vi "RTSystemsCheck (1).vi"(8 "error in":errorcluster) -> (0 "error out":errorcluster)   [LabVIEW 2017]
uses:
  <vilib>/Platform/TimedLoop/XDataNode/timing_clust.ctl
  <vilib>/Platform/TimedLoop/XDataNode/nitl_modes.ctl
  <vilib>/Platform/TimedLoop/XDataNode/wakeup.ctl
  LoopPeriodGLOBAL.vi
  <vilib>/Platform/TimedLoop/XDataNode/loadnilvce.vi
  RTControl/StopGLOBAL.vi
  <vilib>/platform/TimedLoop/XDataNode/XDataNode.xnode
  <vilib>/Platform/TimedLoop/XDataNode/XDNodeRunTimeDep.lvlib
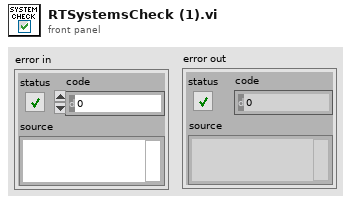
[diagram p1: front panel]
types:
  T1 = typedef "XDNodeRunTimeDep.lvlib/timing_clust.ctl" = cluster{"Expected End [f-1]":u64, "Actual End [f-1]":u64, "Finished Late? [f-1]":bool, "Expected End [i-1]":u64, "Actual End [i-1]":u64, "Finished Late? [i-1]":bool, "Expected Start [i]":u64, "Actual Start [i]":u64, "Expected Start [f]":u64, "Actual Start [f]":u64, "Source Name":string, "Structure Name":string, "Period":i64, "Deadline":i64, "Offset":i64, "Start":i64, "Priority":i32, "Timeout":i32, "Mode":T2, "Wakeup Reason":T3, "Error":errorcluster, "Source Type":string, "Secondary Source Type":string, "Global End Time":u64, "Global Start Time":u64, "Frame Duration":u64, "Iteration Duration":u64, "Assigned CPU":i32, "I/O Scan Engine Mode":u32}
  T2 = typedef "XDNodeRunTimeDep.lvlib/nitl_modes.ctl" = enum32{"No Change", "Process missed periods, maintain original phase", "Discard missed periods, maintain original phase", "Process missed periods, ignore original phase", "Discard missed periods, ignore original phase"}
  T3 = typedef "XDNodeRunTimeDep.lvlib/wakeup.ctl" = enum32{"Normal", "Aborted", "Asynchronous wakeup", "Timing source error", "Timed loop error", "Timeout"}
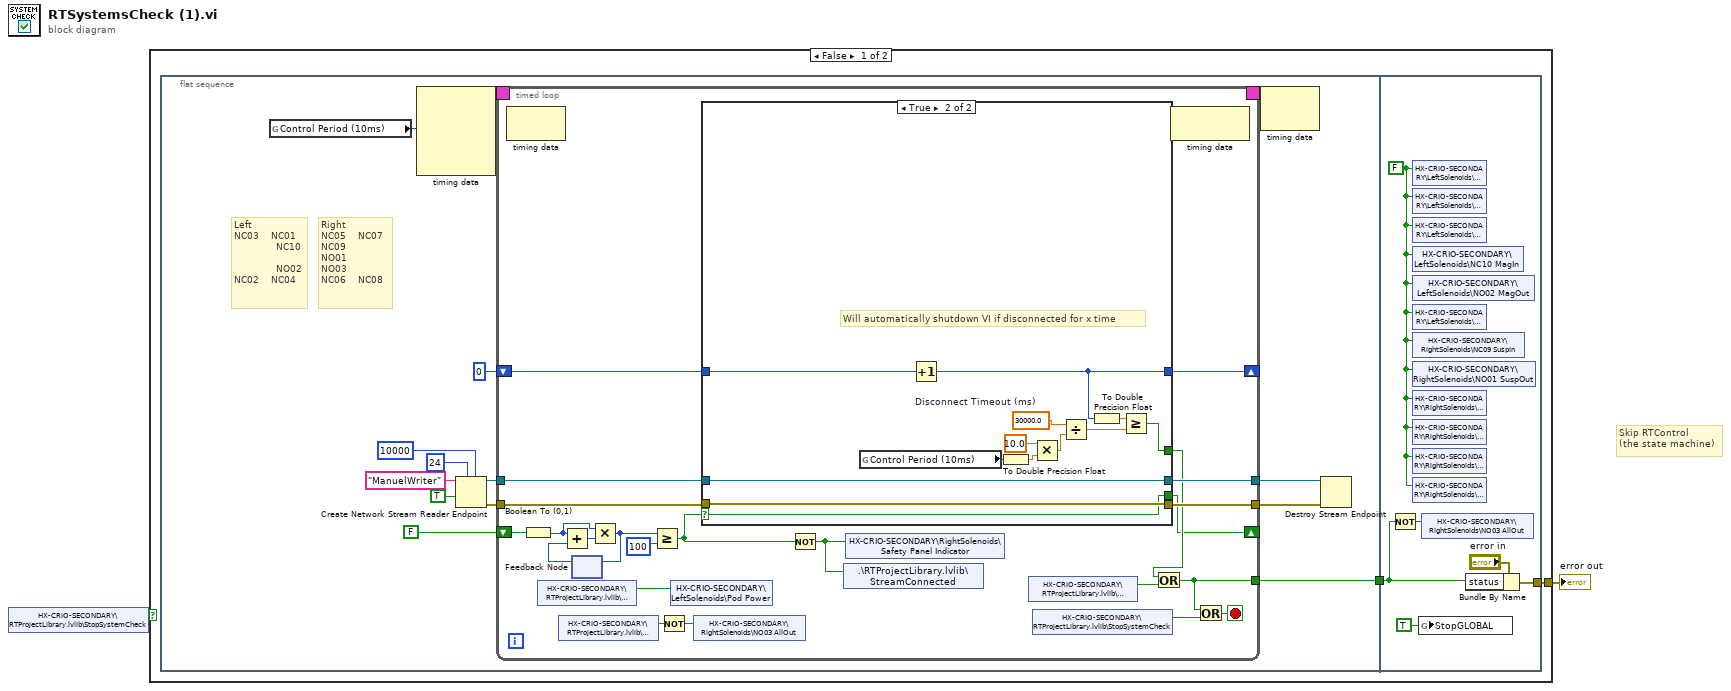
[diagram p0: block diagram]
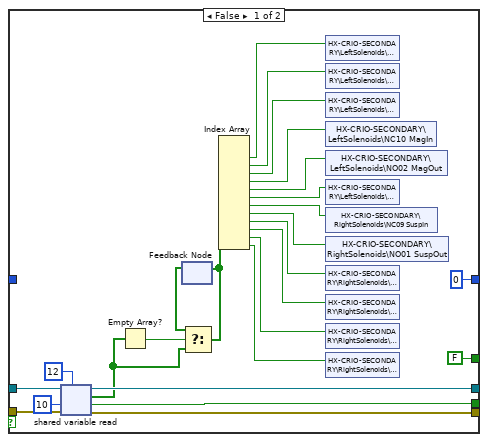
[diagram p2: hidden frame]
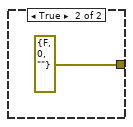
[diagram p3: hidden frame]
diagram:
  # "Skip RTControl\n(the state machine)"
  n1 = shared-variable "HX-CRIO-SECONDARY\\RTProjectLibrary.lvlib\\StopSystemCheck"() -> (w2:bool)  [unwired: 1 in, 1 out]
  n2 = case shown="False" w2 {
    tunnel: [w3 errorcluster {"status"=FALSE, "code"=0, "source"=""} ("error in")] -> w1
    frame False {
      n3 = flat-sequence {
        tunnel: [w7] -> w4
        tunnel: [w89] -> w3
        tunnel: w4 -> [w86]
        frame #0 {
          # "Right\nNC05    NC07\nNC09\nNO01\nNO03\nNC06    NC08"
          # "Left\nNC03    NC01\n              NC10\n\n              NO02\nNC02    NC04"
          n4 = global read "LoopPeriodGLOBAL.vi" "Control Period (10ms)"() -> (w16:i64)
          n5 = node-c288(w16) -> (w18:T1)  [unwired: 3 in]
          n6 = Create Network Stream Reader Endpoint(5:10000 ("timeout in ms (-1)"), 7:24 ("reader buffer size"), 9:TRUE, 11:"ManuelWriter" ("reader name")) -> (0:w14:errorcluster, 3:w15:refnum<k21>)  [unwired: 3 in]
          n7 = timed-loop {
            timing: w18 -> [_]
            timing-out: [_] -> w17
            tunnel: w15 -> [w30]
            tunnel: w14 -> [w29]
            tunnel: [w39] -> w10
            tunnel: [w38] -> w11
            shift-right: [w34] -> _
            shift-left: u16 0 -> [w35]
            tunnel: [w33] -> w7
            shift-right: [w27] -> _
            shift-left: FALSE -> [w25]
            stop <- w40 stop-if-true
            n8 = node-c288() -> ()  [unwired: 1 in, 1 out]
            n9 = Boolean To (0,1)(Boolean=w25) -> (0, 1=w23:i16)
            n10 = shared-variable "HX-CRIO-SECONDARY\\RTProjectLibrary.lvlib\\PodPower"() -> (w28:bool)  [unwired: 1 in, 1 out]
            n11 = shared-variable "HX-CRIO-SECONDARY\\RTProjectLibrary.lvlib\\VentTanks"() -> (w32:bool)  [unwired: 1 in, 1 out]
            n12 = feedback #1() -> (w22:i16)  [unwired: 1 in]
            n13 = Add(x=w23, y=w22) -> (x+y=w24:i16)
            n14 = Multiply(x=w23, y=w24) -> (x*y=w21:i16)
            n15 = feedback-in #1(w21) -> ()
            n16 = Greater Or Equal?(x=w21, y=i16 100) -> (x >= y?=w19:bool)
            n17 = Not(x=w32) -> (.not. x?=w31:bool)
            n18 = shared-variable "HX-CRIO-SECONDARY\\LeftSolenoids\\Pod Power"(w28) -> ()  [unwired: 1 in, 1 out]
            n19 = shared-variable "HX-CRIO-SECONDARY\\RightSolenoids\\NO03 AllOut"(w31) -> ()  [unwired: 1 in, 1 out]
            n20 = case shown="True" w19 {
              selector: w19 -> [_ w67]
              tunnel: [w65 w79] -> w39
              tunnel: [w64 w78] -> w38
              tunnel: w29 -> [w63 w78]
              tunnel: w30 -> [w62 w79]
              tunnel: [FALSE w68] -> w36
              tunnel: w35 -> [_ w77]
              tunnel: [u16 0 w76] -> w34
              tunnel: [w46 w67] -> w27
              frame False {
                n21 = shared-variable-read(w62, w63, 10 ("timeout ms (-1)"), 12 ("# elements")) -> (w65:refnum<k21>, w64:errorcluster, w46:bool, w43:bool[])
                n22 = Empty Array?(array=w43) -> (empty?=w45:bool)
                n23 = feedback #2() -> (w44:bool[])  [unwired: 1 in]
                n24 = Select(t=w44, s=w45, f=w43) -> (s? t:f=w42:bool[])
                n25 = feedback-in #2(w42) -> ()
                n26 = Index Array(array=w42) -> (element #1=w61:bool, element #2=w60:bool, element #3=w59:bool, element #4=w58:bool, element #5=w57:bool, element #6=w56:bool, element #7=w55:bool, element #8=w54:bool, element #9=w53:bool, element #10=w52:bool, element #11=w51:bool, element #12=w50:bool)  [unwired: 12 in]
                n27 = shared-variable "HX-CRIO-SECONDARY\\LeftSolenoids\\NC03"(w61) -> ()  [unwired: 1 in, 1 out]
                n28 = shared-variable "HX-CRIO-SECONDARY\\LeftSolenoids\\NC04"(w60) -> ()  [unwired: 1 in, 1 out]
                n29 = shared-variable "HX-CRIO-SECONDARY\\LeftSolenoids\\NC02"(w59) -> ()  [unwired: 1 in, 1 out]
                n30 = shared-variable "HX-CRIO-SECONDARY\\LeftSolenoids\\NC10 MagIn"(w58) -> ()  [unwired: 1 in, 1 out]
                n31 = shared-variable "HX-CRIO-SECONDARY\\LeftSolenoids\\NO02 MagOut"(w57) -> ()  [unwired: 1 in, 1 out]
                n32 = shared-variable "HX-CRIO-SECONDARY\\LeftSolenoids\\NC01"(w56) -> ()  [unwired: 1 in, 1 out]
                n33 = shared-variable "HX-CRIO-SECONDARY\\RightSolenoids\\NC09 SuspIn"(w55) -> ()  [unwired: 1 in, 1 out]
                n34 = shared-variable "HX-CRIO-SECONDARY\\RightSolenoids\\NO01 SuspOut"(w54) -> ()  [unwired: 1 in, 1 out]
                n35 = shared-variable "HX-CRIO-SECONDARY\\RightSolenoids\\NC08"(w53) -> ()  [unwired: 1 in, 1 out]
                n36 = shared-variable "HX-CRIO-SECONDARY\\RightSolenoids\\NC05"(w52) -> ()  [unwired: 1 in, 1 out]
                n37 = shared-variable "HX-CRIO-SECONDARY\\RightSolenoids\\NC06"(w51) -> ()  [unwired: 1 in, 1 out]
                n38 = shared-variable "HX-CRIO-SECONDARY\\RightSolenoids\\NC07"(w50) -> ()  [unwired: 1 in, 1 out]
              }
              frame True {
                w71 = 30000.0  # Disconnect Timeout (ms)
                # "Will automatically shutdown VI if disconnected for x time"
                n39 = global read "LoopPeriodGLOBAL.vi" "Control Period (10ms)"() -> (w75:i64)
                n40 = Increment(x=w77) -> (x+1=w76:u16)
                n41 = To Double Precision Float(number=w75) -> (double precision float=w74:dbl)
                n42 = Multiply(x=10.0, y=w74) -> (x*y=w73:dbl)
                n43 = Divide(x=w71, y=w73) -> (x/y=w70:dbl)
                n44 = To Double Precision Float(number=w76) -> (double precision float=w69:dbl)
                n45 = Greater Or Equal?(x=w69, y=w70) -> (x >= y?=w68:bool)
              }
            }
            n46 = Not(x=w19) -> (.not. x?=w26:bool)
            n47 = shared-variable ".\\RTProjectLibrary.lvlib\\StreamConnected"(w26) -> ()  [unwired: 1 in, 1 out]
            n48 = shared-variable "HX-CRIO-SECONDARY\\RightSolenoids\\Safety Panel Indicator"(w26) -> ()  [unwired: 1 in, 1 out]
            n49 = shared-variable "HX-CRIO-SECONDARY\\RTProjectLibrary.lvlib\\StopControl"() -> (w37:bool)  [unwired: 1 in, 1 out]
            n50 = shared-variable "HX-CRIO-SECONDARY\\RTProjectLibrary.lvlib\\StopSystemCheck"() -> (w41:bool)  [unwired: 1 in, 1 out]
            n51 = Or(x=w36, y=w37) -> (x .or. y?=w33:bool)
            n52 = node-c288() -> ()  [unwired: 1 in, 1 out]
            n53 = Or(x=w33, y=w41) -> (x .or. y?=w40:bool)
          }
          n54 = node-c288(w17) -> ()  [unwired: 1 out]
          n55 = Destroy Stream Endpoint(8:w11, 11:w10) -> ()  [unwired: 1 out]
        }
        frame #1 {
          w91 = FALSE ("NC03")
          n56 = Not(x=w86) -> (.not. x?=w87:bool)
          n57 = shared-variable "HX-CRIO-SECONDARY\\LeftSolenoids\\NC03"(w91) -> ()  [unwired: 1 in, 1 out]
          n58 = shared-variable "HX-CRIO-SECONDARY\\LeftSolenoids\\NC04"(w91) -> ()  [unwired: 1 in, 1 out]
          n59 = shared-variable "HX-CRIO-SECONDARY\\LeftSolenoids\\NC02"(w91) -> ()  [unwired: 1 in, 1 out]
          n60 = shared-variable "HX-CRIO-SECONDARY\\LeftSolenoids\\NC10 MagIn"(w91) -> ()  [unwired: 1 in, 1 out]
          n61 = shared-variable "HX-CRIO-SECONDARY\\LeftSolenoids\\NO02 MagOut"(w91) -> ()  [unwired: 1 in, 1 out]
          n62 = shared-variable "HX-CRIO-SECONDARY\\LeftSolenoids\\NC01"(w91) -> ()  [unwired: 1 in, 1 out]
          n63 = shared-variable "HX-CRIO-SECONDARY\\RightSolenoids\\NC09 SuspIn"(w91) -> ()  [unwired: 1 in, 1 out]
          n64 = shared-variable "HX-CRIO-SECONDARY\\RightSolenoids\\NO01 SuspOut"(w91) -> ()  [unwired: 1 in, 1 out]
          n65 = shared-variable "HX-CRIO-SECONDARY\\RightSolenoids\\NC08"(w91) -> ()  [unwired: 1 in, 1 out]
          n66 = shared-variable "HX-CRIO-SECONDARY\\RightSolenoids\\NC05"(w91) -> ()  [unwired: 1 in, 1 out]
          n67 = shared-variable "HX-CRIO-SECONDARY\\RightSolenoids\\NC06"(w91) -> ()  [unwired: 1 in, 1 out]
          n68 = shared-variable "HX-CRIO-SECONDARY\\RightSolenoids\\NC07"(w91) -> ()  [unwired: 1 in, 1 out]
          n69 = global write "StopGLOBAL.vi" "StopGLOBAL"(TRUE ("StopGLOBAL")) -> ()
          n70 = shared-variable "HX-CRIO-SECONDARY\\RightSolenoids\\NO03 AllOut"(w87) -> ()  [unwired: 1 in, 1 out]
          n71 = Bundle By Name(cluster="error in", "status"=w86) -> (w89:errorcluster)
        }
      }
    }
    frame True {
    }
  }
  "error out" <- w1
